vi "YAV_90132_Read.vi"(0 "Address":u8, 3 "Drive":enum16{"Phi6", "Simulate", "AtomDrive"}(ring), 5 "error in (no error)":errorcluster) -> (6 "OutputCluster":T1, 7 "Output array":bool[](array[boolean]), 8 "error out":errorcluster)   [LabVIEW 2018]
uses:
  <instrlib>/Phi6/Common/Instrum/Phi6 Core/CANNOU Global Variables.llb/CANNOU Global Variables.gbl.vi
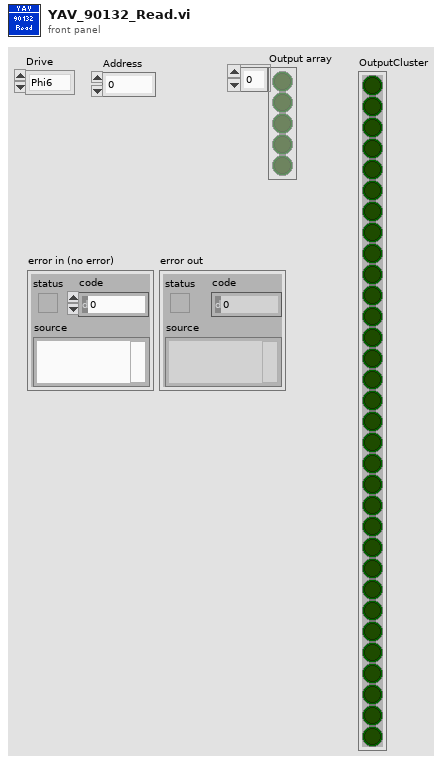
[diagram p1: front panel]
types:
  T1 = cluster{bool, bool, bool, bool, bool, bool, bool, bool, bool, bool, bool, bool, bool, bool, bool, bool, bool, bool, bool, bool, bool, bool, bool, bool, bool, bool, bool, bool, bool, bool, bool, bool}
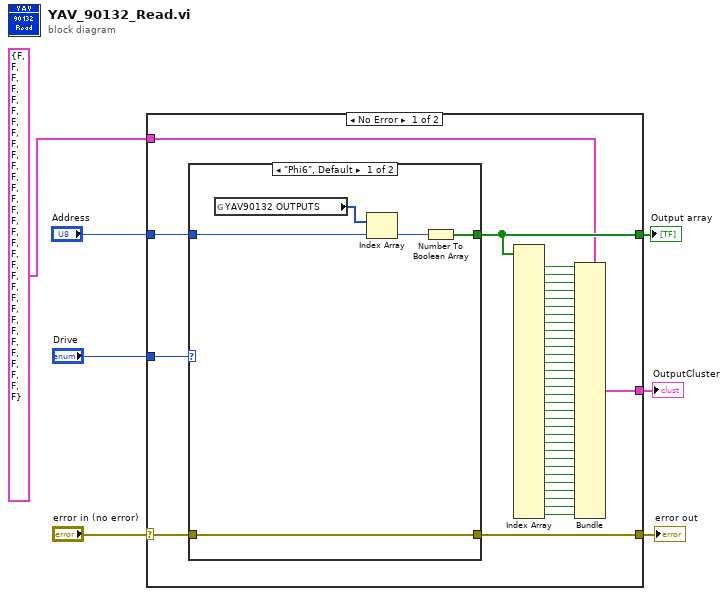
[diagram p0: block diagram]
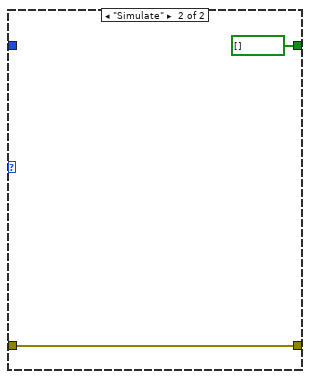
[diagram p2: hidden frame]
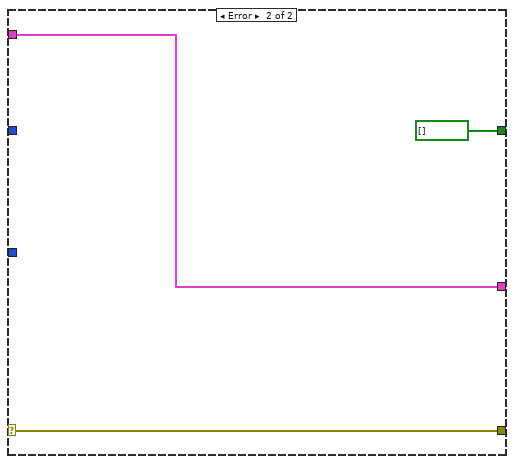
[diagram p3: hidden frame]
diagram:
  n1 = case shown="No Error" "error in (no error)" {
    selector: "error in (no error)" -> [w9 w56]
    tunnel: "Address" -> [w46 _]
    tunnel: [w8 w56] -> w5
    tunnel: [w13 bool[] [] ("Boolean array")] -> w4
    tunnel: [w12 w54] -> w2
    tunnel: T1 {FALSE, FALSE, FALSE, FALSE, FALSE, FALSE, FALSE, FALSE, FALSE, FALSE, FALSE, FALSE, FALSE, FALSE, FALSE, FALSE, FALSE, FALSE, FALSE, FALSE, FALSE, FALSE, FALSE, FALSE, FALSE, FALSE, FALSE, FALSE, FALSE, FALSE, FALSE, FALSE} ("cluster") -> [w11 w54]
    tunnel: "Drive" -> [w10 _]
    frame No Error {
      n2 = case shown="\"Phi6\", Default" w10 {
        tunnel: w46 -> [w50 _]
        tunnel: [w48 bool[] [] ("Boolean array")] -> w13
        tunnel: w9 -> [w47 w52]
        tunnel: [w47 w52] -> w8
        frame "Phi6", Default {
          n3 = global read "CANNOU Global Variables.gbl.vi" "YAV90132 OUTPUTS"() -> (w51:u32[])
          n4 = Index Array(array=w51, index=w50) -> (element=w49:u32)
          n5 = Number To Boolean Array(number=w49) -> (Boolean array=w48:bool[])
        }
        frame "Simulate" {
        }
      }
      n6 = Index Array(array=w13) -> (element #1=w14:bool, element #2=w15:bool, element #3=w16:bool, element #4=w17:bool, element #5=w18:bool, element #6=w19:bool, element #7=w20:bool, element #8=w21:bool, element #9=w22:bool, element #10=w23:bool, element #11=w24:bool, element #12=w25:bool, element #13=w26:bool, element #14=w27:bool, element #15=w28:bool, element #16=w29:bool, element #17=w30:bool, element #18=w31:bool, element #19=w32:bool, element #20=w33:bool, element #21=w34:bool, element #22=w35:bool, element #23=w36:bool, element #24=w37:bool, element #25=w38:bool, element #26=w39:bool, element #27=w40:bool, element #28=w41:bool, element #29=w42:bool, element #30=w43:bool, element #31=w44:bool, element #32=w45:bool)  [unwired: 32 in]
      n7 = Bundle(cluster=w11, w14, w15, w16, w17, w18, w19, w20, w21, w22, w23, w24, w25, w26, w27, w28, w29, w30, w31, w32, w33, w34, w35, w36, w37, w38, w39, w40, w41, w42, w43, w44, w45) -> (w12:T1)
    }
    frame Error {
    }
  }
  "error out" <- w5
  "Output array" <- w4
  "OutputCluster" <- w2
